vi "Parse qSPV Answer.vi"(0 "Answer To Parse":string, 5 "error in":errorcluster) -> (14 "Array of Parameters":T2[](array[typedef]), 19 "error out":errorcluster)   [LabVIEW 2020]
doc: "Parse a SPV? structured answer to a array of parameter sets.\nWill return a warning if some parameters could not be parsed."
uses:
  Parameter Set.ctl
  MemoryType.ctl
  Match Regular Expression.xnode
panel:
  in  "Memory Type":T1
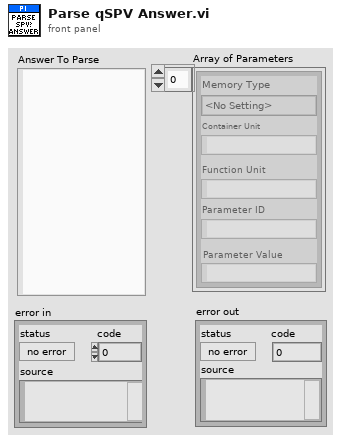
[diagram p1: front panel]
types:
  T1 = typedef "MemoryType.ctl" = enum16{"<No Setting>", "RAM", "FLASH", "TMP"}
  T2 = typedef "Parameter Set.ctl" = cluster{"Memory Type":T1, "Container Unit":string, "Function Unit":string, "Parameter ID":string, "Parameter Value":string}
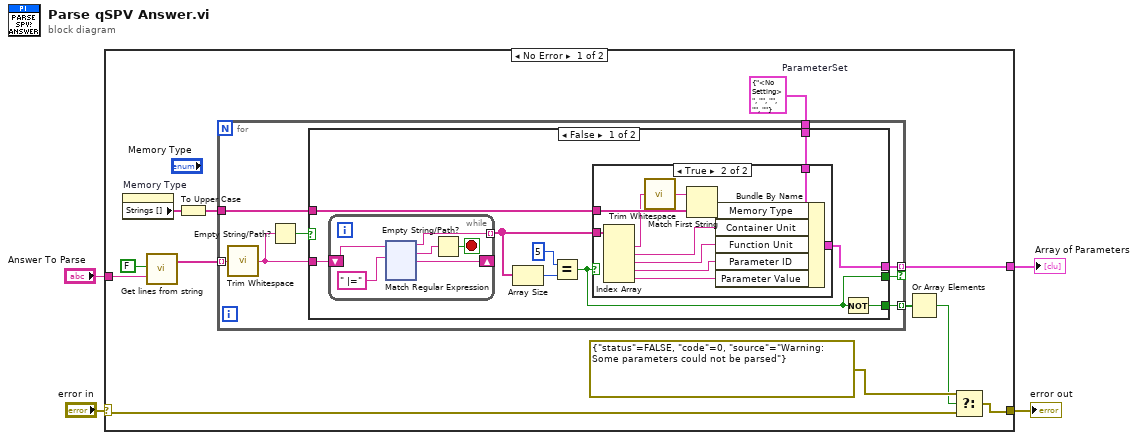
[diagram p0: block diagram]
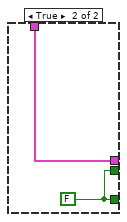
[diagram p3: hidden frame]
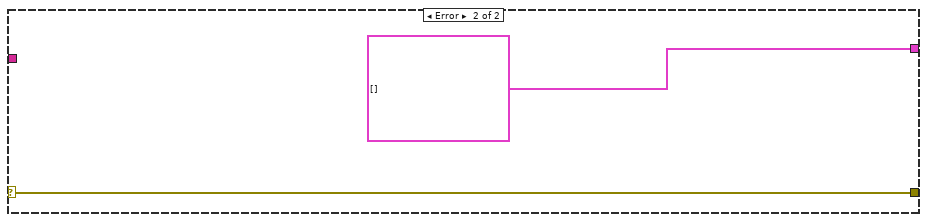
[diagram p4: hidden frame]
diagram:
  n1 = case shown="No Error" "error in" {
    selector: "error in" -> [w5 w168]
    tunnel: "Answer To Parse" -> [w15 _]
    tunnel: [w11 T2[] []] -> w3
    tunnel: [w8 w168] -> w1
    frame No Error {
      w10 = T2 {"Memory Type"=enum."<No Setting>", "Container Unit"="", "Function Unit"="", "Parameter ID"="", "Parameter Value"=""}  # ParameterSet
      n2 = property on="Memory Type" class="Enum (strict)"() -> ("Strings []"=w12:string[])  [unwired: 2 in, 2 out]
      n3 = call "Get lines from string.vi"("Cut spaces?"=FALSE, "Input string"=w15) -> ("Strings"=w14:string[])  [unwired: 16 in, 1 out]
      n4 = To Upper Case(1:w12) -> (0:w13:string[])
      n5 = for {
        tunnel: w14 -> [w24] mode=indexing
        tunnel: w10 -> [w23]
        tunnel: [w22] -> w11 mode=indexing if=w19
        tunnel: w13 -> [w21]
        tunnel: [w20] -> w7 mode=indexing
        n6 = call "Trim Whitespace.vi"("string"=w24) -> ("trimmed string"=w17:string)  [unwired: 1 in]
        n7 = Empty String/Path?(string/path=w17) -> (empty?=w18:bool)
        n8 = case shown="False" w18 {
          tunnel: w23 -> [w33 w166]
          tunnel: [w29 w166] -> w22
          tunnel: w17 -> [w28 _]
          tunnel: w21 -> [w27 _]
          tunnel: [w25 w167] -> w20
          tunnel: [w26 w167] -> w19
          frame False {
            n9 = while {
              shift-right: [w51] -> _
              shift-left: w28 -> [w47]
              tunnel: [w50] -> w30 mode=indexing
              stop <- w48 stop-if-true
              n10 = xnode "Match Regular Expression"("input string"=w47, "regular expression"=" |=") -> ("before match"=w50:string, "whole match"=w49:string, "after match"=w51:string)  [unwired: 4 in, 2 out]
              n11 = Empty String/Path?(string/path=w49) -> (empty?=w48:bool)
            }
            n12 = Array Size(array=w30) -> (size(s)=w32:i32)
            n13 = Equal?(x=5 ("y"), y=w32) -> (x = y?=w26:bool)
            n14 = case shown="True" w26 {
              tunnel: w33 -> [w34 w45]
              tunnel: w30 -> [_ w44]
              tunnel: [w34 w39] -> w29
              tunnel: w27 -> [_ w38]
              frame False {
              }
              frame True {
                n15 = Index Array(array=w44) -> (element #1=w37:string, element #2=w43:string, element #3=w42:string, element #4=w41:string, element #5=w40:string)  [unwired: 5 in]
                n16 = call "Trim Whitespace.vi"("string"=w37) -> ("trimmed string"=w36:string)  [unwired: 1 in]
                n17 = Match First String(2:w38, 3:w36) -> (0:w35:i32)  [unwired: 1 out]
                n18 = Bundle By Name(cluster=w45, "Memory Type"=w35, "Container Unit"=w43, "Function Unit"=w42, "Parameter ID"=w41, "Parameter Value"=w40) -> (w39:T2)
              }
            }
            n19 = Not(x=w26) -> (.not. x?=w25:bool)
          }
          frame True {
            w167 = FALSE
          }
        }
      }
      n20 = Or Array Elements(Boolean array=w7) -> (logical OR=w6:bool)
      n21 = Select(t=errorcluster {"status"=FALSE, "code"=0, "source"="Warning: Some parameters could not be parsed"} ("error in"), s=w6, f=w5) -> (s? t:f=w8:errorcluster)
    }
    frame Error {
    }
  }
  "Array of Parameters" <- w3
  "error out" <- w1
